vi "Dwell.vi"(7 "Points":i32, 10 "Angle":dbl, 11 "Array In":dbl[](array[numeric])) -> (2 "Last Point":dbl, 3 "Array Out":dbl[](array[numeric]))   [LabVIEW 2018]
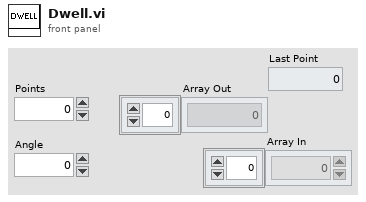
[diagram p1: front panel]
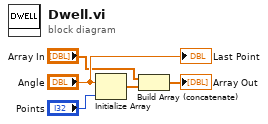
[diagram p0: block diagram]
diagram:
  n1 = Initialize Array("Angle", "Points") -> (w2:dbl[])
  n2 = Build Array (concatenate)("Array In", w2) -> (→"Array Out":dbl[])
  "Last Point" <- "Angle"
